vi "Device Communication Status.vi"(7 "Action?":T4=enum."Get Data", 8 "error in (no error)":errorcluster, 10 "Data":variant, 11 "Device List":T3=enum."Scanner") -> (0 "error out":errorcluster, 3 "Device Status":T1)   [LabVIEW 2021]
uses:
  C/Users/enProducts/Downloads/KIA_Enproducts/KIA_Enproducts/Device Manager/DUT CAN/Controls/DUT Comm Status.ctl
  C/Users/enProducts/Downloads/KIA_Enproducts/KIA_Enproducts/Device Manager/DM Controls/Device Status.ctl
  Gen fgv action.ctl
  C/Users/enProducts/Downloads/KIA_Enproducts/KIA_Enproducts/Device Manager/DM Controls/Device List.ctl
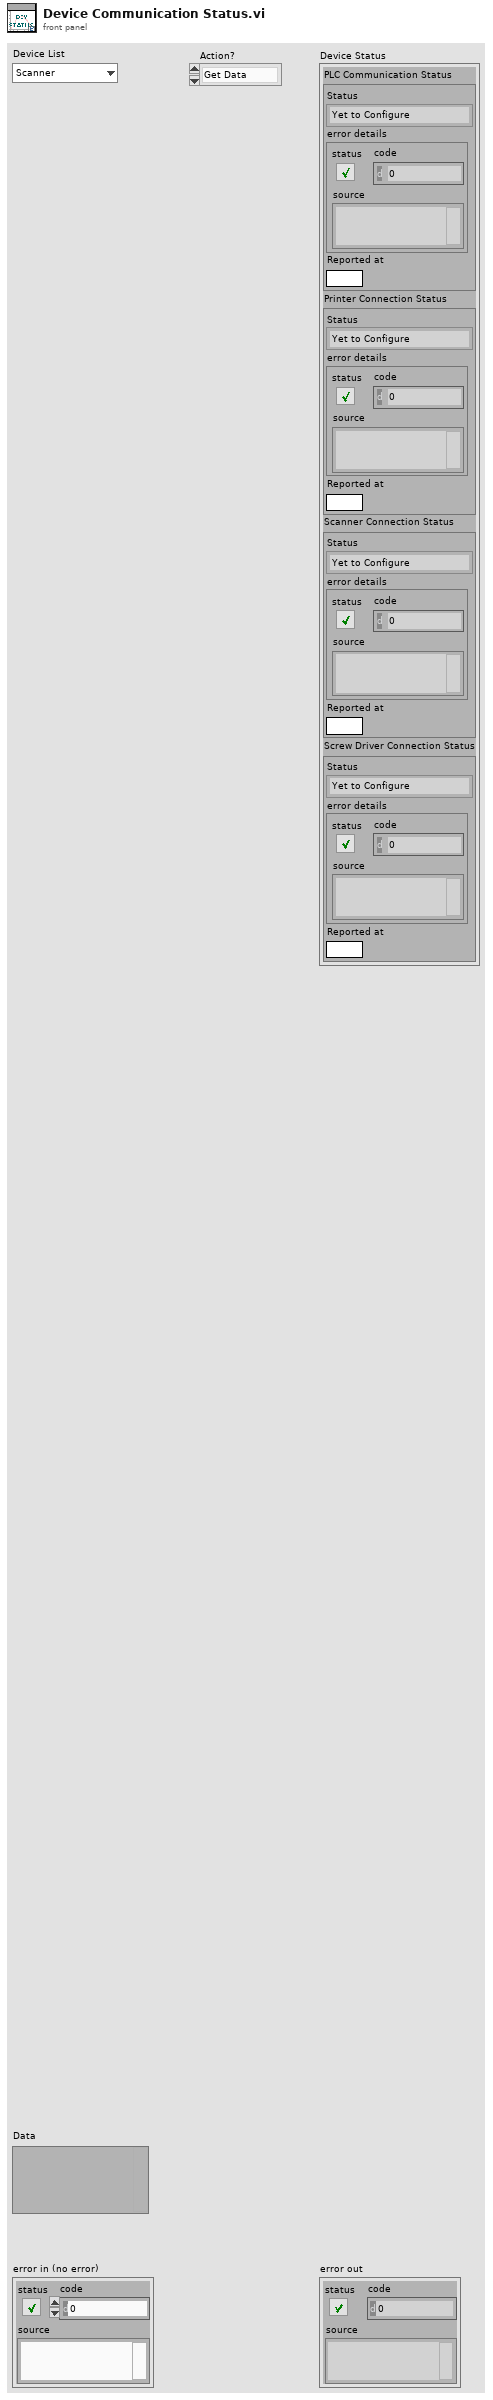
[diagram p1: front panel]
types:
  T1 = typedef "Device Status.ctl" = cluster{"PLC Communication Status":T2, "Printer Connection Status":T2, "Scanner Connection Status":T2, "Screw Driver Connection Status":T2}
  T2 = typedef "DUT Comm Status.ctl" = cluster{"Status":enum16{"Yet to Configure", "Configured", "Connected", "Disconnected", "Error"}, "error details":errorcluster, "Reported at":string}
  T3 = typedef "Device List.ctl" = enum16{"PLC", "Printer", "Scanner", "Screw Driver"}
  T4 = typedef "Gen FGV Action.ctl" = enum16{"Initialize", "Get Data", "Update Data", "Clear Data"}
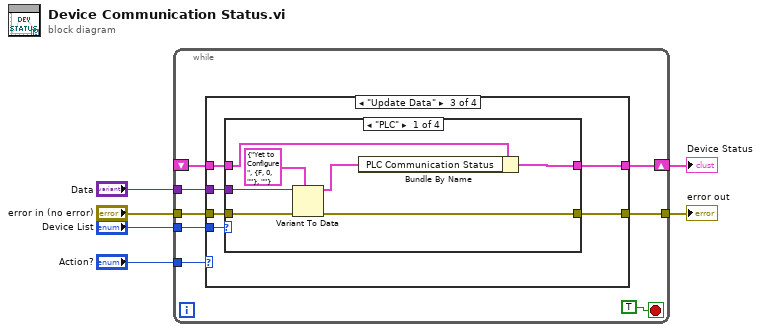
[diagram p0: block diagram]
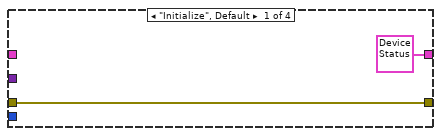
[diagram p2: hidden frame]
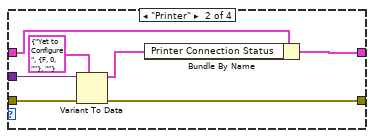
[diagram p4: hidden frame]
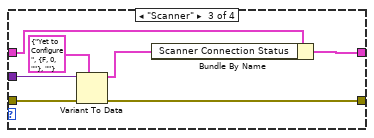
[diagram p5: hidden frame]
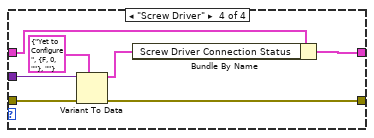
[diagram p6: hidden frame]
diagram:
  n1 = while {
    tunnel: "Action?" -> [w14]
    tunnel: [w7] -> w5
    tunnel: "error in (no error)" -> [w8]
    shift-right: [w12] -> w2
    shift-left: _ -> [w11]
    tunnel: "Device List" -> [w10]
    tunnel: "Data" -> [w9]
    stop <- TRUE stop-if-true
    n2 = case shown="\"Update Data\"" w14 {
      tunnel: [T1 {"PLC Communication Status"={"Status"=enum."Yet to Configure", "error details"={"status"=FALSE, "code"=0, "source"=""}, "Reported at"=""}, "Printer Connection Status"={"Status"=enum."Yet to Configure", "error details"={"status"=FALSE, "code"=0, "source"=""}, "Reported at"=""}, "Scanner Connection Status"={"Status"=enum."Yet to Configure", "error details"={"status"=FALSE, "code"=0, "source"=""}, "Reported at"=""}, "Screw Driver Connection Status"={"Status"=enum."Yet to Configure", "error details"={"status"=FALSE, "code"=0, "source"=""}, "Reported at"=""}} ("Device Status") w18 w23 _] -> w12
      tunnel: w11 -> [_ w18 w22 _]
      tunnel: w10 -> [_ _ w24 _]
      tunnel: w9 -> [_ _ w21 _]
      tunnel: w8 -> [w15 w17 w20 w53]
      tunnel: [w15 w17 w19 w53] -> w7
      frame "Initialize", Default {
      }
      frame "Get Data" {
      }
      frame "Update Data" {
        n3 = case shown="\"PLC\"" w24 {
          tunnel: [w25 w32 w39 w46] -> w23
          tunnel: w22 -> [w27 w34 w41 w48]
          tunnel: w21 -> [w31 w38 w45 w52]
          tunnel: w20 -> [w29 w36 w43 w50]
          tunnel: [w28 w35 w42 w49] -> w19
          frame "PLC" {
            n4 = Variant To Data(error in=w29, type=T2 {"Status"=enum."Yet to Configure", "error details"={"status"=FALSE, "code"=0, "source"=""}, "Reported at"=""} ("DUT Communication Status"), Variant=w31) -> (data=w26:T2, error out=w28:errorcluster)
            n5 = Bundle By Name(cluster=w27, "PLC Communication Status"=w26) -> (w25:T1)
          }
          frame "Printer" {
            n6 = Variant To Data(error in=w36, type=T2 {"Status"=enum."Yet to Configure", "error details"={"status"=FALSE, "code"=0, "source"=""}, "Reported at"=""} ("DUT Communication Status"), Variant=w38) -> (data=w33:T2, error out=w35:errorcluster)
            n7 = Bundle By Name(cluster=w34, "Printer Connection Status"=w33) -> (w32:T1)
          }
          frame "Scanner" {
            n8 = Variant To Data(error in=w43, type=T2 {"Status"=enum."Yet to Configure", "error details"={"status"=FALSE, "code"=0, "source"=""}, "Reported at"=""} ("DUT Communication Status"), Variant=w45) -> (data=w40:T2, error out=w42:errorcluster)
            n9 = Bundle By Name(cluster=w41, "Scanner Connection Status"=w40) -> (w39:T1)
          }
          frame "Screw Driver" {
            n10 = Variant To Data(error in=w50, type=T2 {"Status"=enum."Yet to Configure", "error details"={"status"=FALSE, "code"=0, "source"=""}, "Reported at"=""} ("DUT Communication Status"), Variant=w52) -> (data=w47:T2, error out=w49:errorcluster)
            n11 = Bundle By Name(cluster=w48, "Screw Driver Connection Status"=w47) -> (w46:T1)
          }
        }
      }
      frame "Clear Data" {
      }
    }
  }
  "error out" <- w5
  "Device Status" <- w2
